vi "FP_Close if needed.vi"(8 "Error":errorcluster, 11 "VI":refnum<vi>) -> (0 "Error Out":errorcluster, 3 "VI Out":refnum<vi>)   [LabVIEW 2015]
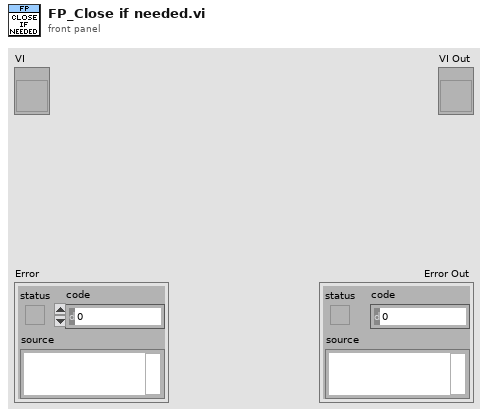
[diagram p1: front panel]
types:
  T1 = enum32{"Invalid", "Standard", "Closed", "Hidden", "Minimized", "Maximized"}
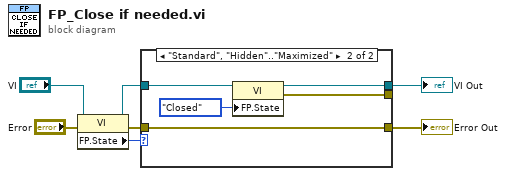
[diagram p0: block diagram]
diagram:
  n1 = property class="VI"(reference="VI", error in="Error") -> (reference out=w3:refnum<vi>, error out=w5:errorcluster, "FP.State"=w7:T1)
  n2 = case shown="\"Standard\", \"Hidden\"..\"Maximized\"" w7 {
    tunnel: w3 -> [w9 w13]
    tunnel: [w9 w12] -> w4
    tunnel: w5 -> [w8 w10]
    tunnel: [w8 w10] -> w6
    tunnel: [_ w11] -> _
    frame "Invalid", "Closed" {
    }
    frame "Standard", "Hidden".."Maximized" {
      n3 = property class="VI"(reference=w13, "FP.State"=T1."Closed" ("Front Panel Window:State")) -> (reference out=w12:refnum<vi>, error out=w11:errorcluster)  [unwired: 1 in]
    }
  }
  "Error Out" <- w6
  "VI Out" <- w4
